vi "fullNameProgram.vi"() -> ()   [LabVIEW 2021]
panel:
  in  "LName":string
  in  "FName":string
  out "Full Name":string
  in  "MName":string
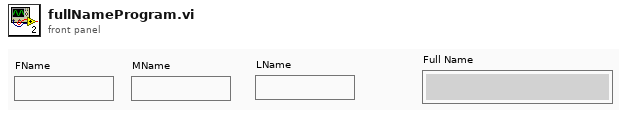
[diagram p1: front panel]
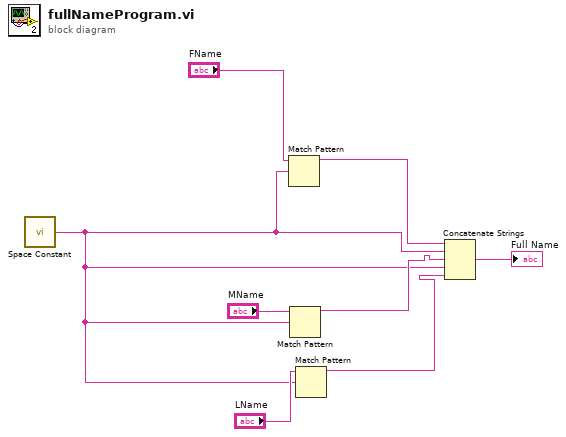
[diagram p0: block diagram]
diagram:
  n1 = call <vilib>:"Space Constant.vi"() -> ("String"=w2:string)
  n2 = Match Pattern(string="FName", regular expression=w2) -> (before substring=w1:string)  [unwired: 1 in, 3 out]
  n3 = Match Pattern(string="MName", regular expression=w2) -> (before substring=w4:string)  [unwired: 1 in, 3 out]
  n4 = Match Pattern(string="LName", regular expression=w2) -> (before substring=w3:string)  [unwired: 1 in, 3 out]
  n5 = Concatenate Strings(w1, w2, w4, w2, w3) -> (→"Full Name":string)
